vi "XML.FindNodeByControl.vi"(8 "error in (no error)":errorcluster, 10 "node in":refnum<k20>, 11 "Control in":refnum<vi>) -> (0 "error out":errorcluster, 1 "found node":refnum<k20>, 2 "node out":refnum<k20>, 3 "Control out":refnum<vi>)   [LabVIEW 2019, in "Tools.lvlib"]
uses:
  Tools.lvlib
  <vilib>/xml/NI_XML.lvlib
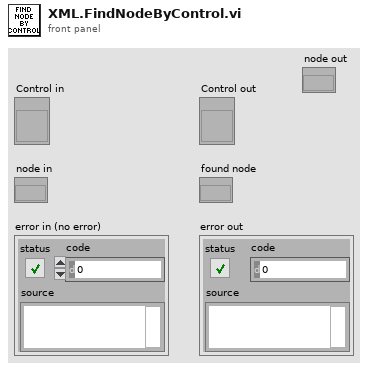
[diagram p1: front panel]
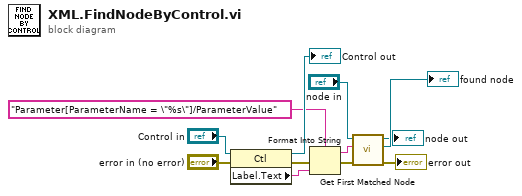
[diagram p0: block diagram]
diagram:
  n1 = property class="Ctl"(reference="Control in", error in="error in (no error)") -> (reference out=→"Control out":refnum<vi>, error out=w8:errorcluster, "Label.Text"=w7:string)
  n2 = Format Into String(format string="Parameter[ParameterName = \"%s\"]/ParameterValue" ("XPath expression"), error in=w8, w7) -> (resulting string=w3:string, error out=w6:errorcluster)  [unwired: 1 in]
  n3 = call <vilib>:"Get First Matched Node.vi"("error in (no error)"=w6, "XPath expression"=w3, "node in"="node in") -> ("error out"=→"error out":errorcluster, "node result"=→"found node":refnum<k20>, "node out"=→"node out":refnum<k20>)  [unwired: 6 in]
